vi "overlaychange.vi"(10 "Angle":dbl=4.0 format="%#_13g", 11 "Bounding Box":cluster{"x":sgl, "y":sgl}[](array[cluster])=[{"x"=467.2217, "y"=730.6483}, {"x"=1215.3674, "y"=677.9415}, {"x"=1227.9468, "y"=856.499}, {"x"=479.80106, "y"=909.2058}, {"x"=467.2217, "y"=730.6483}]) -> (3 "OVERLAYRec":cluster{dbl, dbl, dbl, dbl, "Angle":dbl})   [LabVIEW 2019]
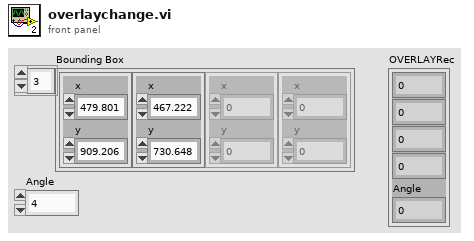
[diagram p1: front panel]
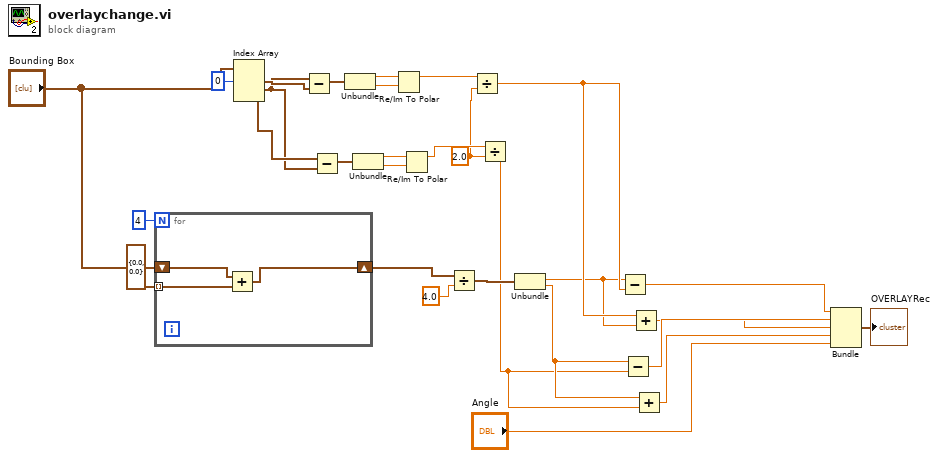
[diagram p0: block diagram]
diagram:
  w17 = sgl 2.0 ("y")
  n1 = for {
    N: 4 -> [_]
    shift-right: [w30] -> w14
    shift-left: cluster{"x":sgl, "y":sgl} {"x"=0.0, "y"=0.0} -> [w32]
    tunnel: "Bounding Box" -> [w31] mode=indexing
    n2 = Add(x=w32, y=w31) -> (x+y=w30:cluster{"x":sgl, "y":sgl})
  }
  n3 = Index Array(array="Bounding Box", index #1=0 ("index")) -> (element #1=w28:cluster{"x":sgl, "y":sgl}, element #2=w20:cluster{"x":sgl, "y":sgl}, element #3=w21:cluster{"x":sgl, "y":sgl})  [unwired: 2 in]
  n4 = Subtract(x=w20, y=w28) -> (x-y=w27:cluster{"x":sgl, "y":sgl})
  n5 = Subtract(x=w21, y=w20) -> (x-y=w22:cluster{"x":sgl, "y":sgl})
  n6 = Unbundle(w27) -> ("x"=w26:sgl, "y"=w25:sgl)
  n7 = Unbundle(w22) -> ("x"=w23:sgl, "y"=w24:sgl)
  n8 = Re/Im To Polar(2:w25, 3:w26) -> (1:w19:sgl)  [unwired: 1 out]
  n9 = Re/Im To Polar(2:w24, 3:w23) -> (1:w18:sgl)  [unwired: 1 out]
  n10 = Divide(x=w14, y=4.0) -> (x/y=w12:cluster{"x":dbl, "y":dbl})
  n11 = Divide(x=w19, y=w17) -> (x/y=w11:sgl)
  n12 = Divide(x=w18, y=w17) -> (x/y=w8:sgl)
  n13 = Unbundle(w12) -> ("x"=w10:dbl, "y"=w9:dbl)
  n14 = Subtract(x=w10, y=w11) -> (x-y=w7:dbl)
  n15 = Subtract(x=w9, y=w8) -> (x-y=w4:dbl)
  n16 = Add(x=w11, y=w10) -> (x+y=w3:dbl)
  n17 = Add(x=w9, y=w8) -> (x+y=w2:dbl)
  n18 = Bundle(w7, w4, w3, w2, "Angle"="Angle") -> (→"OVERLAYRec":cluster{dbl, dbl, dbl, dbl, "Angle":dbl})  [unwired: 1 in]
